vi "Outer_Step.vi"(10 "Sweep States":T1(ring)) -> (3 "AfterAckStep out":T1(ring))   [LabVIEW 2025]
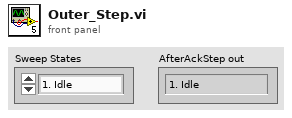
[diagram p1: front panel]
types:
  T1 = enum16{"1. Idle", "2. Start", "3. Apply_Config", "4. Run_Point_Step", "5. Wait ACK", "6. Next Field", "7. Next Temp", "8. Stop"}
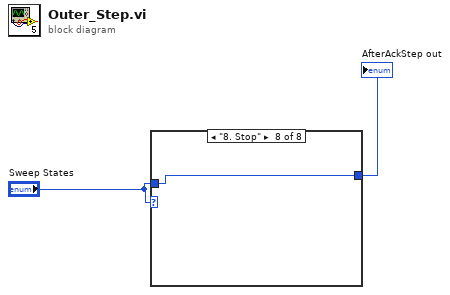
[diagram p0: block diagram]
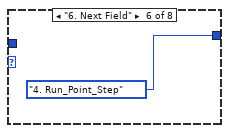
[diagram p7: hidden frame]
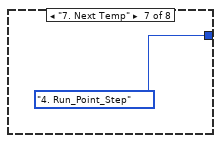
[diagram p8: hidden frame]
diagram:
  n1 = case shown="\"8. Stop\"" "Sweep States" {
    tunnel: [w3 w4 w5 w6 w7 T1."4. Run_Point_Step" ("Sweep States 2") T1."4. Run_Point_Step" ("Sweep States 2") w10] -> w2
    tunnel: "Sweep States" -> [w3 w4 w5 w6 w7 _ _ w10]
    frame "1. Idle", Default {
    }
    frame "2. Start" {
    }
    frame "3. Apply_Config" {
    }
    frame "4. Run_Point_Step" {
    }
    frame "5. Wait ACK" {
    }
    frame "6. Next Field" {
    }
    frame "7. Next Temp" {
    }
    frame "8. Stop" {
    }
  }
  "AfterAckStep out" <- w2
